vi "compute_average_image.vi"(7 "all?":bool, 8 "error in (no error)":errorcluster, 9 "range":i32=1 min=1, 10 "start index":i32 min=0, 11 "ImageCollection in":refnum<class "ImageCollection.lvclass">) -> (0 "error out":errorcluster, 2 "averaged image":refnum<class "Image.lvclass">, 3 "ImageCollection out":refnum<class "ImageCollection.lvclass">)   [LabVIEW 2010, in "ImageCollection.lvclass"]
uses:
  ImageCollection.lvclass
  Image/Image/Image.lvclass
  add_mode_enum.ctl
panel:
  out "size":i32
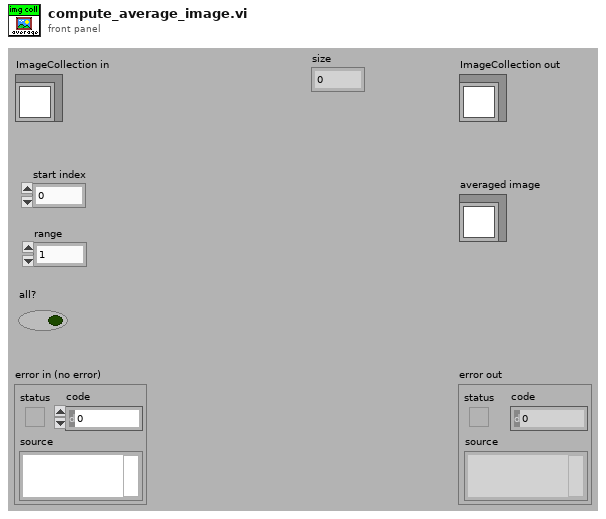
[diagram p1: front panel]
types:
  T1 = typedef "ImageCollection.lvclass/add_mode_enum.ctl" = enum16{"instance", "copy"}
  T2 = typedef "Image Type" = u32
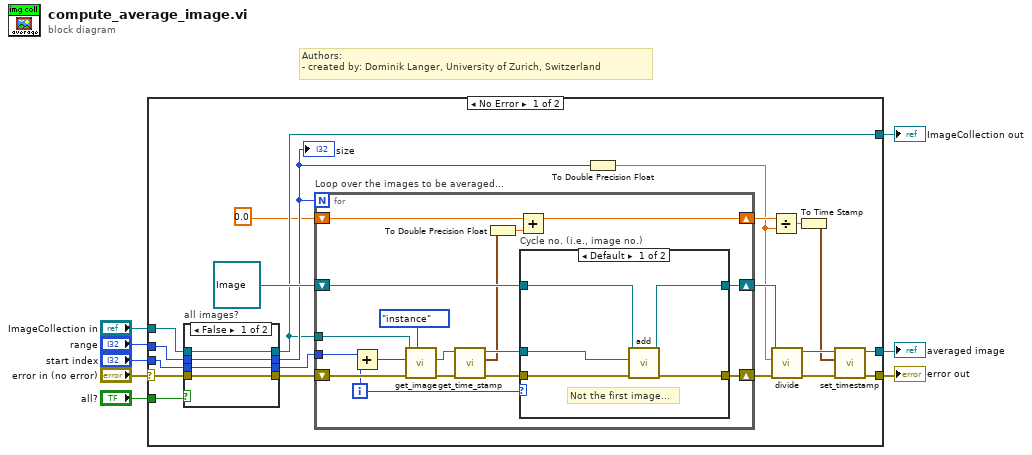
[diagram p0: block diagram]
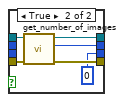
[diagram p2: hidden frame]
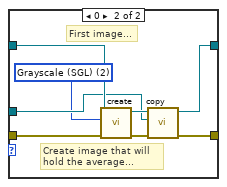
[diagram p3: hidden frame]
diagram:
  # "Authors: \n- created by: Dominik Langer, University of Zurich, Switzerland"
  n1 = case shown="No Error" "error in (no error)" {
    selector: "error in (no error)" -> [w25 w71]
    tunnel: [w10 w71] -> w7
    tunnel: [w20 w70] -> w5
    tunnel: "ImageCollection in" -> [w24 w70]
    tunnel: "start index" -> [w19 _]
    tunnel: "range" -> [w22 _]
    tunnel: [w11 _] -> w2
    tunnel: "all?" -> [w26 _]
    frame No Error {
      n2 = case "all images?" shown="False" w26 {
        tunnel: w25 -> [w33 w39]
        tunnel: w24 -> [w32 w37]
        tunnel: [w33 w38] -> w23
        tunnel: [w32 w36] -> w20
        tunnel: [w31 w34] -> w21
        tunnel: w22 -> [w31 _]
        tunnel: w19 -> [w30 _]
        tunnel: [w30 0 ("start index")] -> w18
        frame False {
        }
        frame True {
          n3 = call-dynamic "get_number_of_images.vi"("error in (no error)"=w39, "ImageCollection in"=w37) -> ("error out"=w38:errorcluster, "size"=w34:i32, "ImageCollection out"=w36:refnum<class "ImageCollection.lvclass">)  [unwired: 7 out]
        }
      }
      "size" <- w21
      n4 = for "Loop over the images to be averaged..." {
        N: w21 -> [_]
        tunnel: w20 -> [w54]
        shift-right: [w52] -> w27
        shift-left: refnum<class "Image.lvclass"> refnum ("Image.lvclass") -> [w53]
        shift-right: [w51] -> w29
        shift-left: w23 -> [w56]
        tunnel: w18 -> [w49]
        shift-right: [w40] -> w16
        shift-left: 0.0 -> [w41]
        i -> [w48]
        n5 = Add(x=w49, y=w48) -> (x+y=w55:i32)
        n6 = call-dynamic "get_image.vi"("get image as..."=add_mode_enum."instance", "error in (no error)"=w56, "index"=w55, "ImageCollection in"=w54) -> ("error out"=w47:errorcluster, "Image.lvclass"=w46:refnum<class "Image.lvclass">)  [unwired: 6 out]
        n7 = call-dynamic "get_time_stamp.vi"("error in (no error)"=w47, "Image.lvclass in"=w46) -> ("error out"=w44:errorcluster, "timestamp"=w43:timestamp, "Image.lvclass out"=w45:refnum<class "Image.lvclass">)  [unwired: 7 out]
        n8 = To Double Precision Float(number=w43) -> (double precision float=w42:dbl)
        n9 = Add(x=w41, y=w42) -> (x+y=w40:dbl)
        n10 = case "Cycle no. (i.e., image no.)" shown="Default" w48 {
          tunnel: w53 -> [w60 w67]
          tunnel: w44 -> [w61 w65]
          tunnel: w45 -> [w59 w64]
          tunnel: [w57 w62] -> w52
          tunnel: [w58 w69] -> w51
          frame Default {
            # "Not the first image..."
            n11 = call-dynamic "add.vi"("error in (no error)"=w61, "addend"=w59, "Image in"=w60) -> ("error out"=w58:errorcluster, "Image out"=w57:refnum<class "Image.lvclass">)  [unwired: 1 in, 6 out]
          }
          frame 0 {
            w63 = T2 2 items=["Grayscale (U8)", "Grayscale (I16)", "Grayscale (SGL)", "Complex (CSG)", "RGB (U32)", "HSL (U32)", "RGB (U64)", "Grayscale (U16)"] ("Image Type")
            # "First image..."
            # "Create image that will hold the average..."
            n12 = call "create.vi"("error in (no error)"=w65, "Image Type"=w63, "Image in"=w67) -> ("error out"=w68:errorcluster, "Image out"=w66:refnum<class "Image.lvclass">)  [unwired: 1 in, 6 out]
            n13 = call "copy.vi"("error in (no error)"=w68, "image to copy (source)"=w64, "Image in (target)"=w66) -> ("error out"=w69:errorcluster, "Image out"=w62:refnum<class "Image.lvclass">)  [unwired: 7 out]
          }
        }
      }
      n14 = To Double Precision Float(number=w21) -> (double precision float=w9:dbl)
      n15 = Divide(x=w16, y=w9) -> (x/y=w15:dbl)
      n16 = call-dynamic "divide.vi"("error in (no error)"=w29, "divisor"=w9, "Image in"=w27) -> ("error out"=w14:errorcluster, "Image out"=w13:refnum<class "Image.lvclass">)  [unwired: 1 in, 6 out]
      n17 = To Time Stamp(1:w15) -> (0:w12:timestamp)
      n18 = call-dynamic "set_timestamp.vi"("error in (no error)"=w14, "timestamp"=w12, "Image.lvclass in"=w13) -> ("error out"=w10:errorcluster, "Image.lvclass out"=w11:refnum<class "Image.lvclass">)  [unwired: 7 out]
    }
    frame Error {
    }
  }
  "error out" <- w7
  "ImageCollection out" <- w5
  "averaged image" <- w2
